vi "ET3500 - Write Registers.vi"(4 "Simulate":bool, 5 "ET3500 Segment Enum":T2 items=["Segment.Type", "Segment.Holdback", "", "", "Segment.Duration", "Segment.RampRate", "Segment.TargetSP", "Segment.EndAction", "", "", "", "", "", "", "", "", "Segment.GsoakType", "Segment.GsoakVal"], 6 "Option":cluster{"Init":bool, "Close":bool}={"Init"=TRUE, "Close"=TRUE}, 7 "ET3500 Programmer Enum":T1 items=["Comms.ProgramNumber", "", "Program.RampUnits", "Program.DwellUnits", "", "", "", "", "", "Programmer.CurProg", "Programmer.CurSeg", "Programmer.ProgStatus", "", "", "", "", "", "Programmer.ProgTimeLeft", "Programmer.PVIn", "Programmer.SPIn", "", "Programmer.SegTimeLeft"], 8 "error in (no error)":errorcluster, 9 "Process Variable  (0)":i32=1, 10 "ET3500 Enum":T3, 11 "VISA resource name":refnum<visa-resource-name>="COM3") -> (0 "error out":errorcluster, 3 "VISA resource name out":refnum<visa-resource-name>)   [LabVIEW 2013]
uses:
  Controls/ET3500 Enum.ctl
  Controls/ET3500 Segment Enum.ctl
  Controls/ET3500 Programmer Enum.ctl
  <instrlib>/Eurotherm 35xx Series/Eurotherm 35xx Series.lvlib
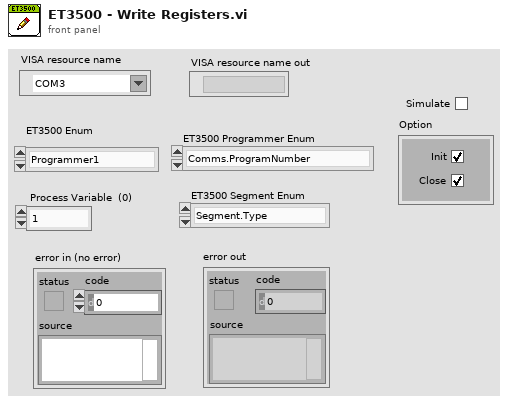
[diagram p1: front panel]
types:
  T1 = typedef "ET3500 Programmer Enum.ctl" = u16
  T2 = typedef "ET3500 Segment Enum.ctl" = u16
  T3 = typedef "ET3500 Enum.ctl" = enum16{"Programmer1", "Segment1", "Segment2", "Segment3", "Segment4", "Segment5", "Segment6", "Segment7", "Segment8", "Segment9", "Segment10", "Segment11", "Segment12", "Segment13", "Segment14", "Segment15", "Segment16"}
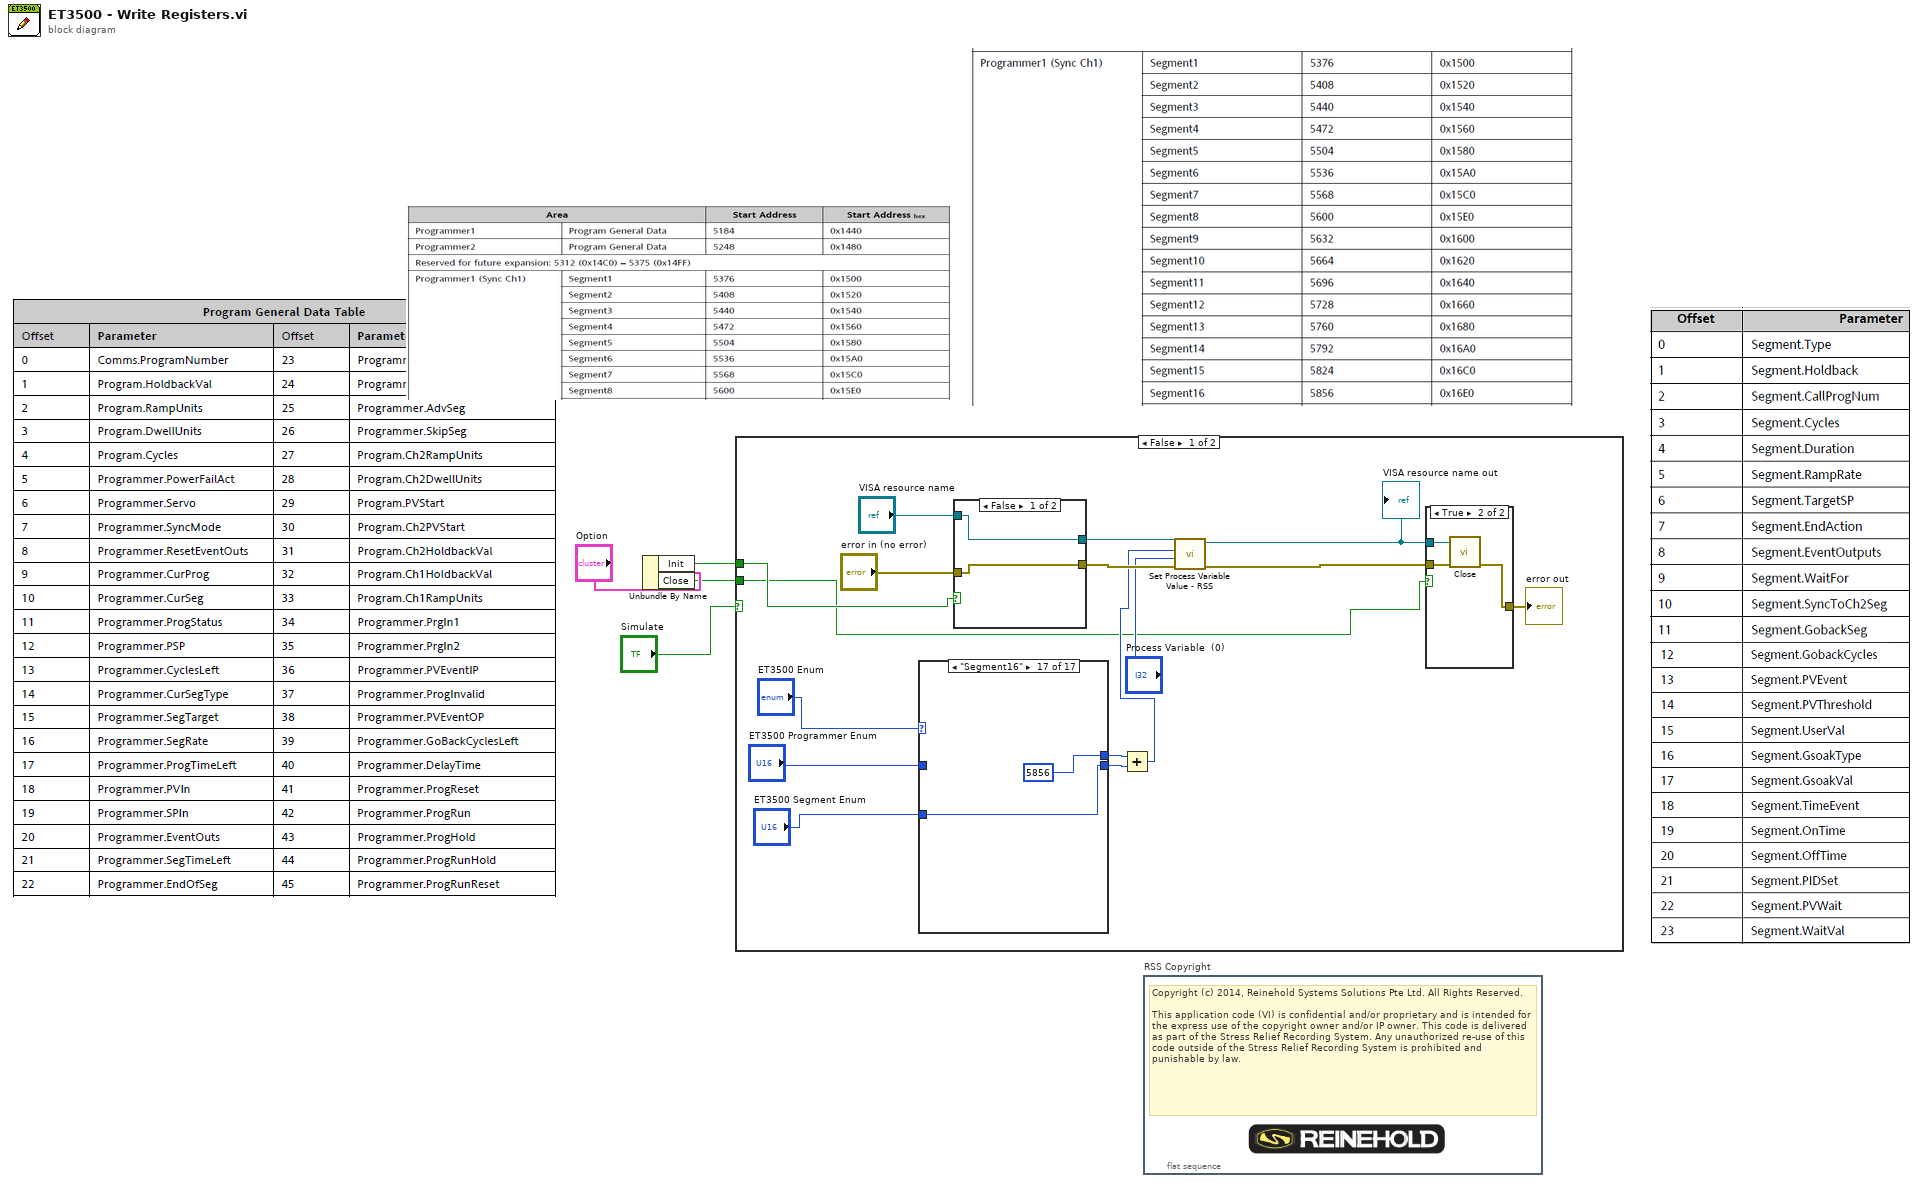
[diagram p0: block diagram]
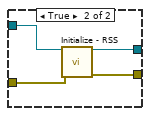
[diagram p3: hidden frame]
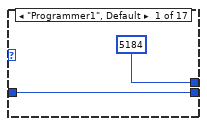
[diagram p4: hidden frame]
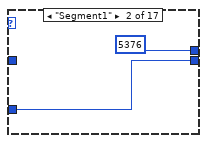
[diagram p5: hidden frame]
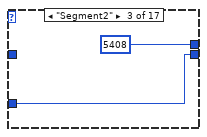
[diagram p6: hidden frame]
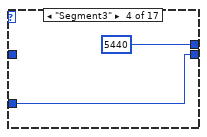
[diagram p7: hidden frame]
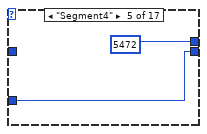
[diagram p8: hidden frame]
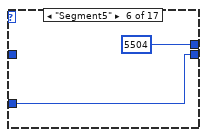
[diagram p9: hidden frame]
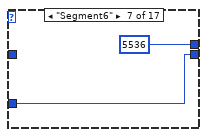
[diagram p10: hidden frame]
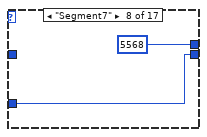
[diagram p11: hidden frame]
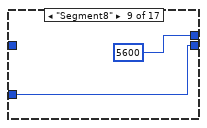
[diagram p12: hidden frame]
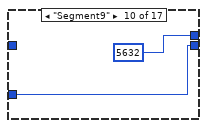
[diagram p13: hidden frame]
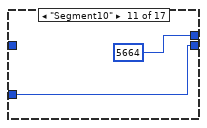
[diagram p14: hidden frame]
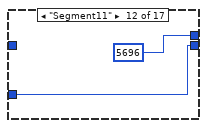
[diagram p15: hidden frame]
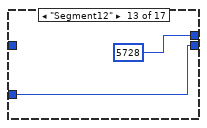
[diagram p16: hidden frame]
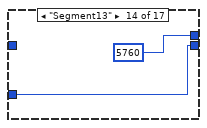
[diagram p17: hidden frame]
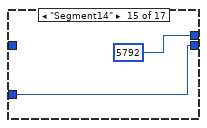
[diagram p18: hidden frame]
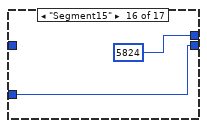
[diagram p19: hidden frame]
diagram:
  n1 = Unbundle By Name("Option") -> ("Init"=w3:bool, "Close"=w2:bool)
  n2 = case shown="False" "Simulate" {
    tunnel: w3 -> [w6 _]
    tunnel: w2 -> [w5 _]
    frame False {
      n3 = case shown="\"Segment16\"" "ET3500 Enum" {
        tunnel: "ET3500 Programmer Enum" -> [w31 _ _ _ _ _ _ _ _ _ _ _ _ _ _ _ _]
        tunnel: [u16 5184 ("Register Address (0)") u16 5376 ("Register Address (0)") u16 5408 ("Register Address (0)") u16 5440 ("Register Address (0)") u16 5472 ("Register Address (0)") u16 5504 ("Register Address (0)") u16 5536 ("Register Address (0)") u16 5568 ("Register Address (0)") u16 5600 ("Register Address (0)") u16 5632 ("Register Address (0)") u16 5664 ("Register Address (0)") u16 5696 ("Register Address (0)") u16 5728 ("Register Address (0)") u16 5760 ("Register Address (0)") u16 5792 ("Register Address (0)") u16 5824 ("Register Address (0)") u16 5856 ("Register Address (0)")] -> w11
        tunnel: [w31 w33 w35 w37 w40 w41 w44 w46 w48 w50 w52 w54 w56 w58 w60 w62 w64] -> w10
        tunnel: "ET3500 Segment Enum" -> [_ w33 w35 w37 w40 w41 w44 w46 w48 w50 w52 w54 w56 w58 w60 w62 w64]
        frame "Programmer1", Default {
        }
        frame "Segment1" {
        }
        frame "Segment2" {
        }
        frame "Segment3" {
        }
        frame "Segment4" {
        }
        frame "Segment5" {
        }
        frame "Segment6" {
        }
        frame "Segment7" {
        }
        frame "Segment8" {
        }
        frame "Segment9" {
        }
        frame "Segment10" {
        }
        frame "Segment11" {
        }
        frame "Segment12" {
        }
        frame "Segment13" {
        }
        frame "Segment14" {
        }
        frame "Segment15" {
        }
        frame "Segment16" {
        }
      }
      n4 = case shown="False" w6 {
        tunnel: "VISA resource name" -> [w26 w30]
        tunnel: [w25 w29] -> w19
        tunnel: [w26 w28] -> w18
        tunnel: "error in (no error)" -> [w25 w27]
        frame False {
        }
        frame True {
          n5 = call <instrlib>:"Initialize - RSS.vi"("VISA resource name"=w30, "error in (no error)"=w27) -> ("VISA resource name out"=w28:refnum<visa-resource-name>, "error out"=w29:errorcluster)  [unwired: 12 in]
        }
      }
      n6 = Add(x=w11, y=w10) -> (x+y=w8:T2)
      n7 = call "Set Process Variable Value - RSS.vi"("error in (no error)"=w19, "Process Variable  (0)"="Process Variable  (0)", "Register Addresses (0)"=w8, "VISA resource name"=w18) -> ("error out"=w17:errorcluster, "VISA resource name out"=w16:refnum<visa-resource-name>)  [unwired: 6 in]
      "VISA resource name out" <- w16
      n8 = case shown="True" w5 {
        tunnel: w17 -> [w21 w24]
        tunnel: w16 -> [_ w23]
        tunnel: [w21 w22] -> w14
        frame False {
        }
        frame True {
          n9 = call <instrlib>:"Close.vi"("VISA resource name"=w23, "error in (no error)"=w24) -> ("error out"=w22:errorcluster)  [unwired: 13 in]
        }
      }
      "error out" <- w14
    }
    frame True {
    }
  }
  n10 = flat-sequence "RSS Copyright" {
    frame #0 {
      # "Copyright (c) 2014, Reinehold Systems Solutions Pte Ltd. All Rights Reserved.\n\nThis application code (VI) is confidential and/or proprietary and is intended for the express use of the copyright owner and/or IP owner. This code is delivered as part of the Stress Relief Recording System. Any unauthorized re-use of this code outside of the Stress Relief Recording System is prohibited and punishable by law."
    }
  }
